vi "Flatten I32.vi"(3 "I32":i32, 4 "Endian":T1) -> (5 "Flat Data":u8[](array[numeric]) format="%.0x")   [LabVIEW 2021, in "DataTypes_CIF_U.lvlib"]
uses:
  Endian.ctl
  DataTypes_CIF_U.lvlib
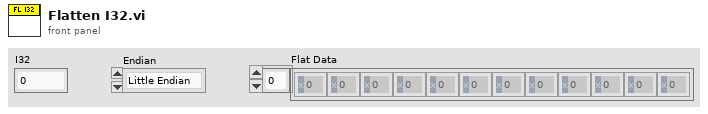
[diagram p1: front panel]
types:
  T1 = typedef "DataTypes_CIF_U.lvlib/Endian.ctl" = enum16{"Little Endian", "Big Endian"}
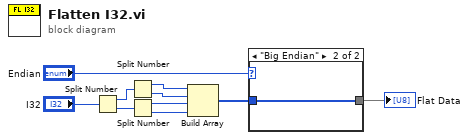
[diagram p0: block diagram]
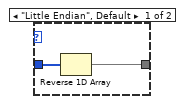
[diagram p2: hidden frame]
diagram:
  n1 = Split Number(x="I32") -> (hi(x)=w1:u16, lo(x)=w5:u16)
  n2 = Split Number(x=w1) -> (hi(x)=w2:u8, lo(x)=w3:u8)
  n3 = Split Number(x=w5) -> (hi(x)=w4:u8, lo(x)=w6:u8)
  n4 = Build Array(w2, w3, w4, w6) -> (w10:u8[])
  n5 = case shown="\"Big Endian\"" "Endian" {
    tunnel: w10 -> [w12 w13]
    tunnel: [w11 w13] -> w8
    frame "Little Endian", Default {
      n6 = Reverse 1D Array(array=w12) -> (reversed array=w11:u8[])
    }
    frame "Big Endian" {
    }
  }
  "Flat Data" <- w8
